vi "Wait on Message.vi"(8 "error in (no error)":errorcluster, 11 "ConnectionReader in":refnum<class "ConnectionReader.lvclass">) -> (0 "error out":errorcluster, 2 "Self Enqueuer":refnum<class "Message Enqueuer.lvclass">, 3 "ConnectionReader out":refnum<class "ConnectionReader.lvclass">)   [LabVIEW 2019, in "ConnectionReader.lvlib" / "ConnectionReader.lvclass"]
uses:
  <vilib>/gpm_packages/@cs/Network-interface/Source/ConnectionReader/ConnectionReader/ConnectionReader.lvclass
  C:/Program Files/National Instruments/LabVIEW 2019/vi.lib/gpm_packages/@cs/Network-interface/Source/Logged Actor/LoggedActor.lvclass
  C:/Program Files/National Instruments/LabVIEW 2019/vi.lib/ActorFramework/Actor/Actor.lvclass
  <vilib>/ActorFramework/Message Enqueuer/Message Enqueuer.lvclass
  <vilib>/gpm_packages/@cs/Network-interface/Source/ConnectionReader/ConnectionReader/ConnectionReader.lvclass/ConnectionReader.ctl
  <vilib>/gpm_packages/@cs/Network-interface/Source/MessagingInterfaces/IPacket/IPacket.lvclass
  <vilib>/gpm_packages/@cs/event-logger/Source/Composed Log/Types/Log Level.ctl
  <vilib>/gpm_packages/@cs/Network-interface/Source/Logged Actor/LoggedActor.lvclass/LoggedActor.ctl
  <vilib>/gpm_packages/@cs/event-logger/Source/Composed Log/LoggerReference/LoggerReference.lvclass/LoggerReference.ctl
  <vilib>/ActorFramework/Actor/Actor.lvclass/Actor.ctl
  <vilib>/ActorFramework/Message Enqueuer/Message Enqueuer.lvclass/Message Enqueuer.ctl
  <vilib>/gpm_packages/@cs/event-logger/Source/Composed Log/LoggerReference/Log Event.vi
  <vilib>/ActorFramework/Message Enqueuer/Init from Existing Queue.vi
  <vilib>/gpm_packages/@cs/event-logger/Source/Composed Log/LoggerReference/Log.vi
  <vilib>/gpm_packages/@cs/event-logger/Source/Composed Log/LoggerReference/Get Valid Event Time.vi
  <vilib>/gpm_packages/@cs/event-logger/Source/Composed Log/LoggerReference/Remove Stale Logs.vi
  <vilib>/gpm_packages/@cs/Network-interface/Source/MessagingInterfaces/IReadStrategy/IReadStrategy.lvclass
  <vilib>/gpm_packages/@cs/Network-interface/Source/MessagingInterfaces/IMessageReturnPolicy/IMessageReturnPolicy.lvclass
  <vilib>/ActorFramework/Actor/Actor.lvclass
  <vilib>/gpm_packages/@cs/Network-interface/Source/Logged Actor/LoggedActor.lvclass
  <vilib>/gpm_packages/@cs/event-logger/Source/Composed Log/Composed Log.lvlib
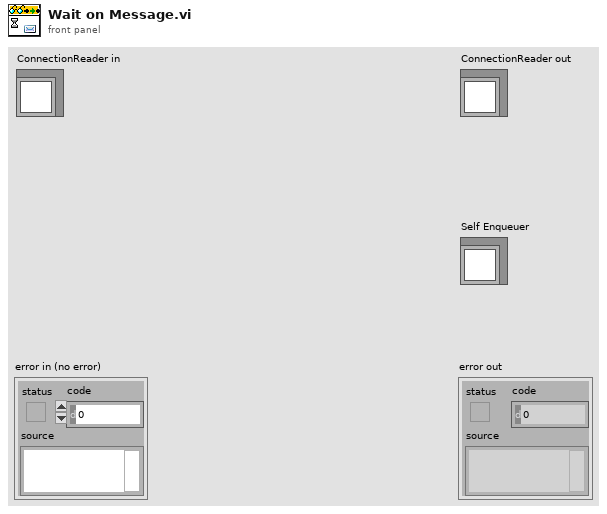
[diagram p1: front panel]
types:
  T1 = typedef "Composed Log.lvlib/Log Level.ctl" = enum16{"Debug", "Info", "Warning", "Error", "Critical"}
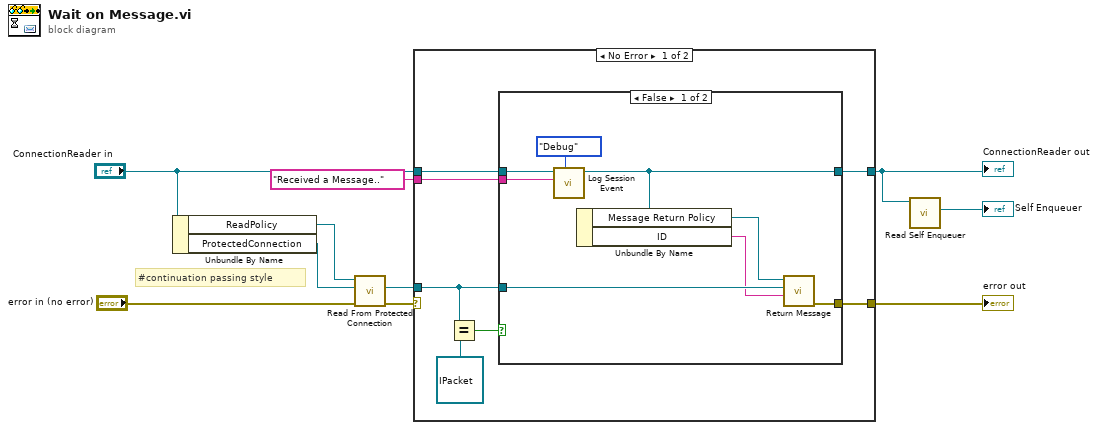
[diagram p0: block diagram]
diagram:
  # "#continuation passing style"
  n1 = Unbundle By Name("ConnectionReader in") -> ("ReadPolicy"=w9:refnum<class "IReadStrategy.lvclass">, "ProtectedConnection"=w6:refnum<class "ProtectedConnectionReader.lvclass">)
  n2 = call-dynamic "Read From Protected Connection.vi"("error in (no error)"="error in (no error)", "ProtectedConnectionReader"=w6, "IReadPolicy in"=w9) -> ("error out"=w8:errorcluster, "Packet"=w5:refnum<class "IPacket.lvclass">)  [unwired: 7 in]
  n3 = case shown="No Error" w8 {
    selector: w8 -> [_ w27]
    tunnel: "ConnectionReader in" -> [w15 w28]
    tunnel: [w14 w28] -> w1
    tunnel: [w12 w27] -> w10
    tunnel: w5 -> [w17 _]
    tunnel: "Received a Message.." ("Event Data") -> [w11 _]
    frame No Error {
      n4 = Equal?(x=w17, y=refnum<class "IPacket.lvclass"> refnum) -> (x = y?=w13:bool)
      n5 = case shown="False" w13 {
        tunnel: w17 -> [w25 _]
        tunnel: w15 -> [w24 w26]
        tunnel: [w21 w26] -> w14
        tunnel: [w22 _] -> w12
        tunnel: w11 -> [w19 _]
        frame False {
          n6 = call <vilib>:"Log Session Event.vi"("Event Level"=Log_Level."Debug", "Event Data"=w19, "SessionActor in"=w24) -> ("SessionActor out"=w21:refnum<class "ConnectionReader.lvclass">)  [unwired: 7 in, 1 out]
          n7 = Unbundle By Name(w21) -> ("Message Return Policy"=w23:refnum<class "IMessageReturnPolicy.lvclass">, "ID"=w18:string)
          n8 = call-dynamic "Return Message.vi"("Connection ID"=w18, "Message To Return"=w25, "IMessageReturnPolicy in"=w23) -> ("error out"=w22:errorcluster)  [unwired: 8 in]
        }
        frame True {
        }
      }
    }
    frame Error {
    }
  }
  "error out" <- w10
  "ConnectionReader out" <- w1
  n9 = call <vilib>:"Read Self Enqueuer.vi"("Actor"=w1) -> ("Self Enqueuer"=→"Self Enqueuer":refnum<class "Message Enqueuer.lvclass">)  [unwired: 10 in]
